vi "Configuration Page.vi"(8 "Error In":errorcluster, 11 "Sample Test Template in":refnum<class "Sample Test Template.lvclass">) -> (0 "Error Out":errorcluster, 3 "Sample Test Template out":refnum<class "Sample Test Template.lvclass">)   [LabVIEW 2020, in "Sample Test Template.lvclass"]
doc: "Configuration page Template"
uses:
  Sample Test Template.lvclass
  Typedef/User event controls.ctl
  ADC DAC Test Measurement.lvlib
panel:
  # "Sample Configuration page"
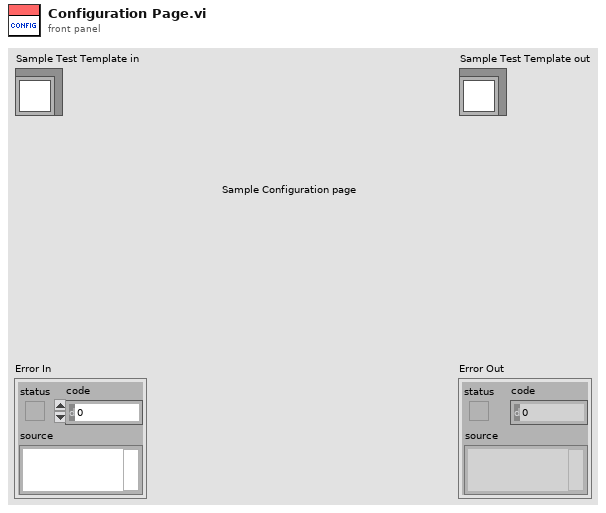
[diagram p1: front panel]
types:
  T1 = typedef "ADC DAC Test Measurement.lvlib/User event controls.ctl" = enum16{"Create", "Generate", "Run Test", "Get Ref", "Destroy"}
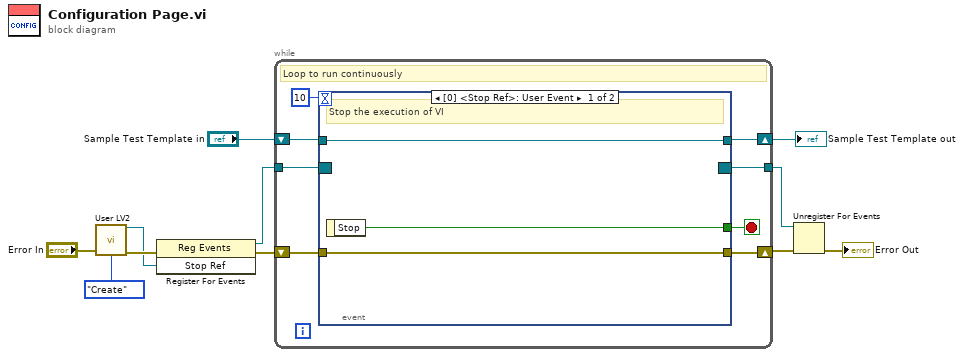
[diagram p0: block diagram]
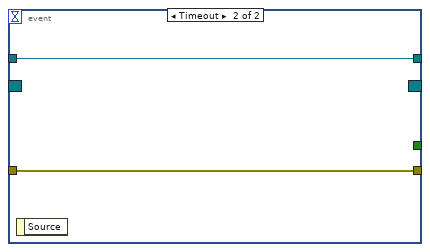
[diagram p2: hidden frame]
diagram:
  n1 = call "User LV2.vi"("Error In"="Error In", "User event controls"=User_event_controls."Create") -> ("Stop Ref"=w9:refnum<user-event>, "Error Out"=w10:errorcluster)  [unwired: 11 in, 1 out]
  n2 = register-events(error in=w10, w9) -> (reference out=w8:refnum<event-registration>, error out=w7:errorcluster)  [unwired: 1 in]
  n3 = while {
    tunnel: w8 -> [w19]
    shift-right: [w17] -> w1
    shift-left: "Sample Test Template in" -> [w18]
    shift-right: [w14] -> w6
    shift-left: w7 -> [w15]
    tunnel: [w13] -> w5
    stop <- w16 stop-if-true
    # "Loop to run continuously"
    n4 = event shown="[0] <Stop Ref>: User Event" {
      selector: w19 -> [_ _]
      dyn-events: [_ _] -> w13
      timeout: 10 -> [_ _]
      tunnel: [w20 w23] -> w17
      tunnel: w18 -> [w20 w23]
      tunnel: [w22 _] -> w16
      tunnel: w15 -> [w21 w24]
      tunnel: [w21 w24] -> w14
      event User Event {
        # "Stop the execution of VI"
        n5 = event-data() -> ("Stop"=w22:bool)  [unwired: 1 in]
      }
      event Timeout {
        n6 = event-data() -> ()  [unwired: 1 in, 1 out]
      }
    }
  }
  "Sample Test Template out" <- w1
  n7 = Unregister For Events(event registration refnum=w5, error in=w6) -> (error out=→"Error Out":errorcluster)
